vi "FTDI SPI SYS Read.vi"(6 "nCS":u8 max=4 step=1, 7 "ClockRate":u32=50000, 8 "Use Extra":bool, 10 "Addr":T1 items=["Addr-0", "Addr-1", "Addr-2", "Addr-3", "Addr-4", "Addr-5", "Addr-6", "Addr-7"], 11 "Handler In":u32) -> (0 "error out":errorcluster, 1 "Out Reg B Bin":bool[](array[boolean]), 2 "Out Reg A Bin":bool[](array[boolean]), 3 "Handler Out":u32, 4 "Out Reg B Dec":u16, 5 "Out Reg A Dec":u16)   [LabVIEW 2018]
uses:
  PROJEKT/NIKO/Labview/Niko V4/FTDI SPI/Ctl/Sub Addr.ctl
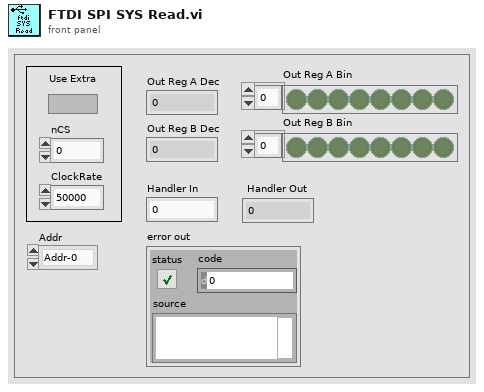
[diagram p1: front panel]
types:
  T1 = typedef "Sub Addr.ctl" = u16
  T2 = cluster{"ClockRate":u32, "LatencyTimer":u8, "configOptions 24-31":i8, "configOptions 16-23":i8, "configOptions 8-15":i8, "configOptions 0-7":u32, "Pin":u32, "reserved":u16}
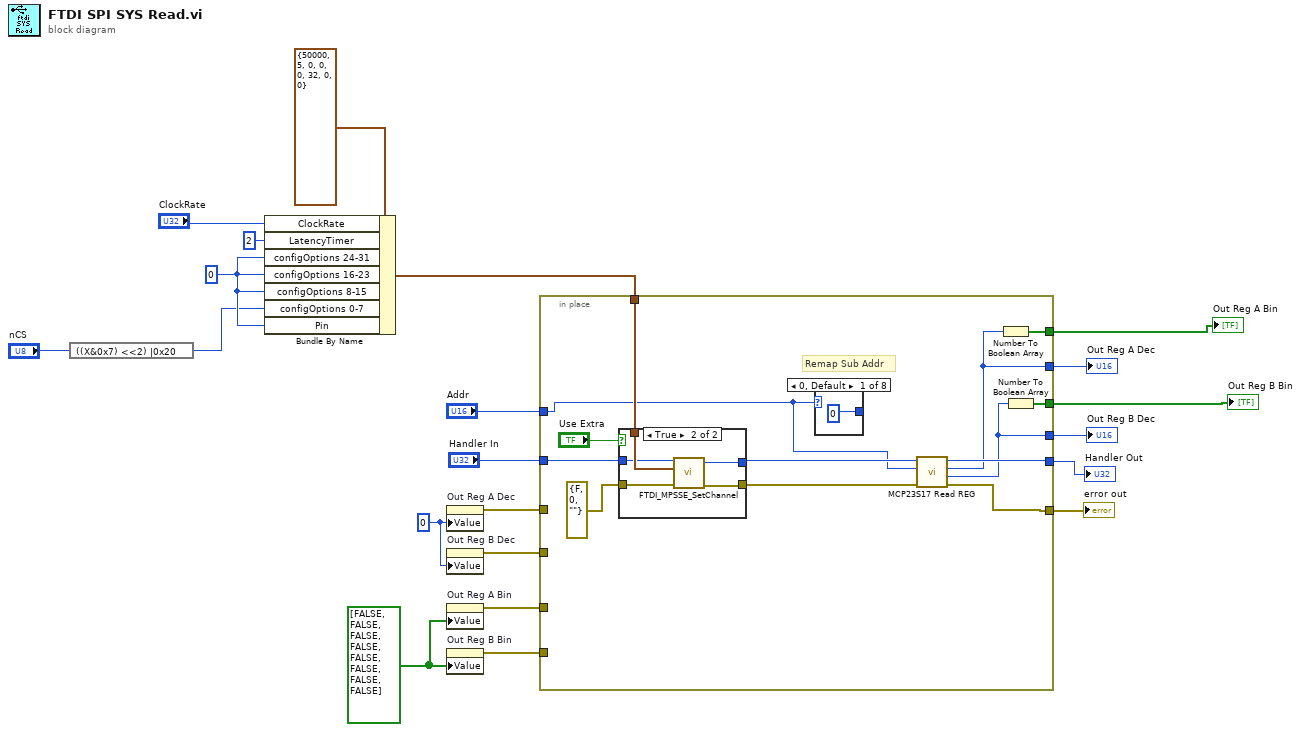
[diagram p0: block diagram]
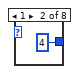
[diagram p2: hidden frame]
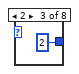
[diagram p3: hidden frame]
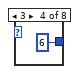
[diagram p4: hidden frame]
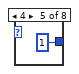
[diagram p5: hidden frame]
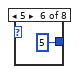
[diagram p6: hidden frame]
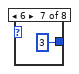
[diagram p7: hidden frame]
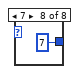
[diagram p8: hidden frame]
diagram:
  w4 = bool[] [FALSE, FALSE, FALSE, FALSE, FALSE, FALSE, FALSE, FALSE] ("Out Reg A Bin")
  w14 = i8 0 ("configOptions 16-23")
  w6 = u16 0 ("LATCH Reg")
  n1 = expression code="((X&0x7) <<2) |0x20"("nCS") -> (w12:u8)
  n2 = Bundle By Name(cluster=T2 {"ClockRate"=50000, "LatencyTimer"=5, "configOptions 24-31"=0, "configOptions 16-23"=0, "configOptions 8-15"=0, "configOptions 0-7"=32, "Pin"=0, "reserved"=0} ("config"), "ClockRate"="ClockRate", "LatencyTimer"=u8 2, "configOptions 24-31"=w14, "configOptions 16-23"=w14, "configOptions 8-15"=w14, "configOptions 0-7"=w12, "Pin"=w14) -> (w17:T2)
  n3 = property on="Out Reg A Dec" class="DigNum (strict)"("Value"=w6) -> (error out=w10:errorcluster)  [unwired: 2 in, 1 out]
  n4 = property on="Out Reg B Dec" class="DigNum (strict)"("Value"=w6) -> (error out=w7:errorcluster)  [unwired: 2 in, 1 out]
  n5 = property on="Out Reg A Bin" class="Arr (strict)"("Value"=w4) -> (error out=w5:errorcluster)  [unwired: 2 in, 1 out]
  n6 = property on="Out Reg B Bin" class="Arr (strict)"("Value"=w4) -> (error out=w3:errorcluster)  [unwired: 2 in, 1 out]
  n7 = in-place {
    in-place-border: [w28] -> w21
    in-place-border: [w27] -> w20
    in-place-border: "Handler In" -> [w34]
    in-place-border: [w26] -> w8
    in-place-border: "Addr" -> [w22]
    in-place-border: w17 -> [w33]
    in-place-border: w10 -> [_]
    in-place-border: [w24] -> w9
    in-place-border: [w25] -> w2
    in-place-border: [w23] -> w1
    in-place-border: w7 -> [_]
    in-place-border: w5 -> [_]
    in-place-border: w3 -> [_]
    # "Remap Sub Addr"
    n8 = case shown="True" "Use Extra" {
      tunnel: w34 -> [w44 w45]
      tunnel: [w44 w48] -> w30
      tunnel: [w43 w49] -> w29
      tunnel: errorcluster {"status"=FALSE, "code"=0, "source"=""} ("error constant") -> [w43 w47]
      tunnel: w33 -> [_ w46]
      frame False {
      }
      frame True {
        n9 = call "FTDI_MPSSE_SetChannel.vi"("error in (no error)"=w47, "config"=w46, "handle"=w45) -> ("error out"=w49:errorcluster, "handle out"=w48:u32)  [unwired: 7 in]
      }
    }
    n10 = case shown="0, Default" w22 {
      tunnel: [0 4 2 6 1 5 3 7] -> _
      frame 0, Default {
      }
      frame 1 {
      }
      frame 2 {
      }
      frame 3 {
      }
      frame 4 {
      }
      frame 5 {
      }
      frame 6 {
      }
      frame 7 {
      }
    }
    n11 = call "MCP23S17 Read REG.vi"("error in (no error)"=w29, "Addr"=w22, "handle"=w30) -> ("error out"=w27:errorcluster, "REG B"=w24:u16, "REG A"=w26:u16, "handle out"=w28:u32)  [unwired: 3 in, 2 out]
    n12 = Number To Boolean Array(number=w26) -> (Boolean array=w25:bool[])
    n13 = Number To Boolean Array(number=w24) -> (Boolean array=w23:bool[])
  }
  "Handler Out" <- w21
  "error out" <- w20
  "Out Reg A Dec" <- w8
  "Out Reg A Bin" <- w2
  "Out Reg B Dec" <- w9
  "Out Reg B Bin" <- w1
